vi "Configure Standard Waveform.vi"(4 "DC Offset (0.00 V)":dbl, 6 "Amplitude Units (Vpp)":u16(ring) items=["Vpp", "Vrms", "dBm"], 7 "Frequency (1000 Hz)":dbl=1000.0, 8 "error in (no error)":errorcluster, 9 "Amplitude (1.0 Vpp)":dbl=1.0, 10 "Waveform Function (0: Sine)":u16(ring) items=["Sine", "Square", "Triangle", "Cosine", "DC", "Positive Ramp", "Negative Ramp", "Haversine", "Havercosine", "Sine (x)/x"], 11 "VISA resource name":refnum<visa-resource-name>) -> (0 "error out":errorcluster, 3 "VISA resource name out":refnum<visa-resource-name>)   [LabVIEW 2015, in "Fluke 28x Series.lvlib"]
doc: "Selects the waveform shape, frequency, amplitude, offset, and phase for a standard waveform."
uses:
  <instrlib>/Fluke 28x Series/Fluke 28x Series.lvlib
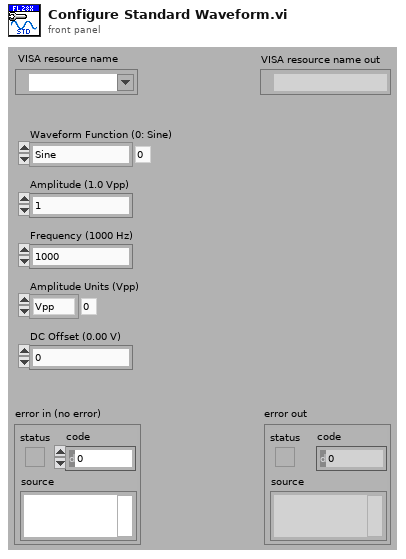
[diagram p1: front panel]
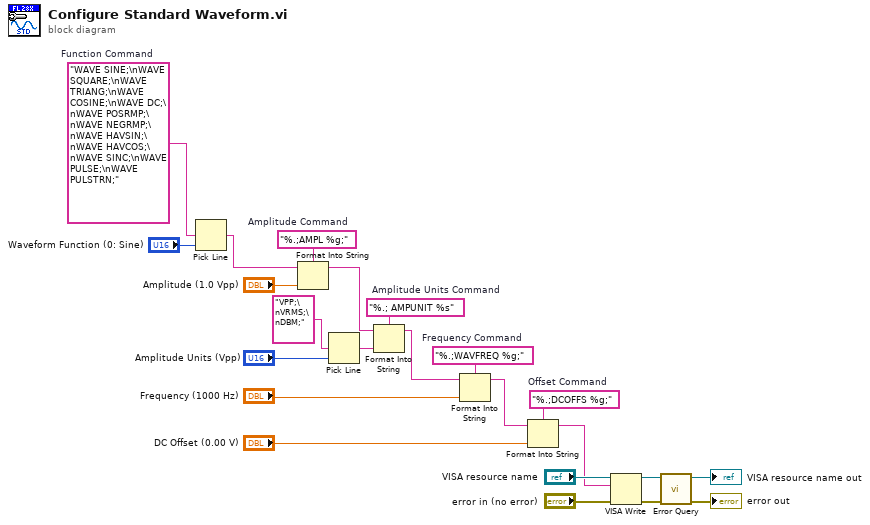
[diagram p0: block diagram]
diagram:
  w8 = "%.; AMPUNIT %s"  # Amplitude Units Command
  w15 = "%.;DCOFFS %g;"  # Offset Command
  w11 = "%.;AMPL %g;"  # Amplitude Command
  w12 = "%.;WAVFREQ %g;"  # Frequency Command
  w16 = "WAVE SINE;\nWAVE SQUARE;\nWAVE TRIANG;\nWAVE COSINE;\nWAVE DC;\nWAVE POSRMP;\nWAVE NEGRMP;\nWAVE HAVSIN;\nWAVE HAVCOS;\nWAVE SINC;\nWAVE PULSE;\nWAVE PULSTRN;"  # Function Command
  n1 = Pick Line(multi-line string=w16, line index="Waveform Function (0: Sine)") -> (output string=w1:string)  [unwired: 1 in]
  n2 = Format Into String(format string=w11, initial string=w1, "Amplitude (1.0 Vpp)") -> (resulting string=w7:string)  [unwired: 1 in, 1 out]
  n3 = Pick Line(multi-line string="VPP;\nVRMS;\nDBM;", line index="Amplitude Units (Vpp)") -> (output string=w5:string)  [unwired: 1 in]
  n4 = Format Into String(format string=w8, initial string=w7, w5) -> (resulting string=w6:string)  [unwired: 1 in, 1 out]
  n5 = Format Into String(format string=w12, initial string=w6, "Frequency (1000 Hz)") -> (resulting string=w13:string)  [unwired: 1 in, 1 out]
  n6 = Format Into String(format string=w15, initial string=w13, "DC Offset (0.00 V)") -> (resulting string=w2:string)  [unwired: 1 in, 1 out]
  n7 = VISA Write(VISA resource name="VISA resource name", write buffer=w2, error in (no error)="error in (no error)") -> (VISA resource name out=w19:refnum<visa-resource-name>, error out=w18:errorcluster)  [unwired: 1 out]
  n8 = call <instrlib>:"Error Query.vi"("error in (no error)"=w18, "VISA resource name"=w19) -> ("error out"=→"error out":errorcluster, "VISA resource name out"=→"VISA resource name out":refnum<visa-resource-name>)  [unwired: 6 in, 2 out]
